vi "Set.vi"(6 "Compliance":dbl, 9 "Voltage":dbl, 10 "SMU":dbl, 11 "VISA Refnum in":refnum<visa-resource-name>) -> (3 "VISA Refnum out":refnum<visa-resource-name>)   [LabVIEW 2022 SP3]
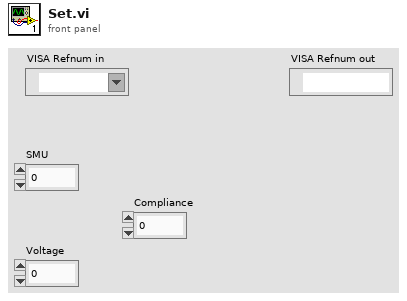
[diagram p1: front panel]
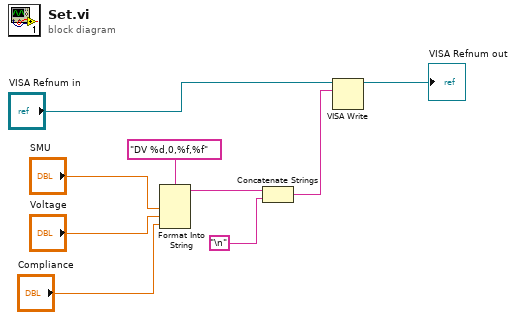
[diagram p0: block diagram]
diagram:
  n1 = Format Into String(format string="DV %d,0,%f,%f", "SMU", "Voltage", "Compliance") -> (resulting string=w6:string)  [unwired: 2 in, 1 out]
  n2 = Concatenate Strings(w6, "\n") -> (w8:string)
  n3 = VISA Write(VISA resource name="VISA Refnum in", write buffer=w8) -> (VISA resource name out=→"VISA Refnum out":refnum<visa-resource-name>)  [unwired: 1 in, 2 out]
